vi "New Data Point.vi"(8 "error in (no error)":errorcluster, 10 "X":dbl format="%#_13g", 11 "Data Generator in":refnum<class "Data Generator.lvclass">) -> (0 "error out":errorcluster, 2 "Y(X)":dbl, 3 "Data Generator out":refnum<class "Data Generator.lvclass">)   [LabVIEW 2020, in "Interfaces.lvlib" / "Data Generator.lvclass"]
uses:
  Data Generator.lvclass
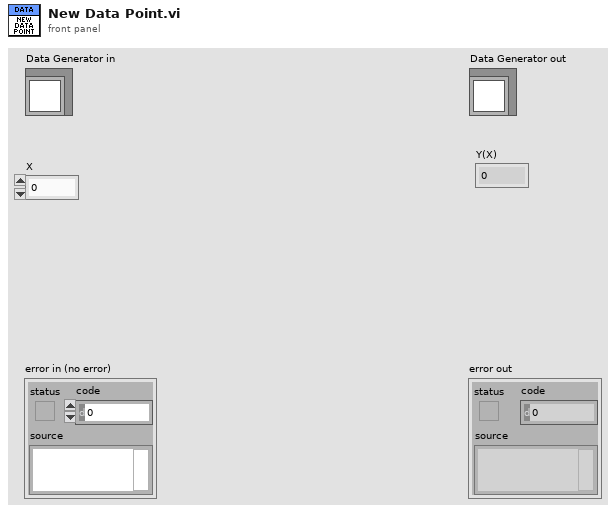
[diagram p1: front panel]
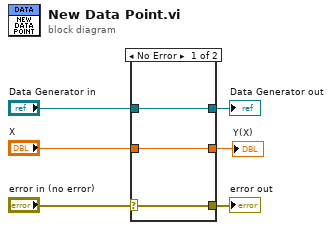
[diagram p0: block diagram]
diagram:
  n1 = case shown="No Error" "error in (no error)" {
    selector: "error in (no error)" -> [w8 w11]
    tunnel: [w8 w11] -> w5
    tunnel: [w9 w10] -> w3
    tunnel: "Data Generator in" -> [w9 w10]
    tunnel: [w7 _] -> w2
    tunnel: "X" -> [w7 _]
    frame No Error {
    }
    frame Error {
    }
  }
  "error out" <- w5
  "Data Generator out" <- w3
  "Y(X)" <- w2
